vi "AttributeElementToString.vi"(8 "error in (no error)":errorcluster, 10 "attributeElement":T1, 11 "WriteAttribute in":refnum<class "XMLAttributeGenerator.lvclass">) -> (0 "error out":errorcluster, 2 "AttributeString":string, 3 "WriteAttribute out":refnum<class "XMLAttributeGenerator.lvclass">)   [LabVIEW 2016, in "XML.lvlib" / "XMLAttributeGenerator.lvclass"]
doc: "This method calls the format attribute method for a single attribute."
uses:
  <userlib>/Common/XML/XMLAttributeGenerator/XMLAttributeGenerator.lvclass
  <userlib>/Common/XML/Typedefs/AttributeElements.ctl
  <vilib>/dlg_ctls.llb/Space Constant.vi
  <userlib>/Common/XML/XML.lvlib
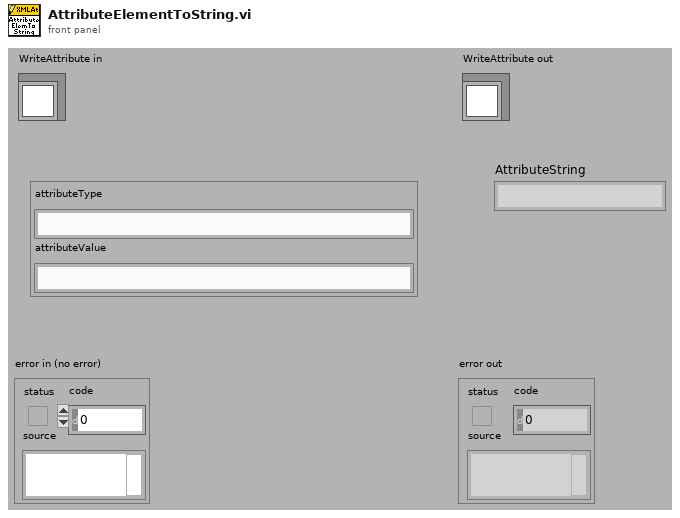
[diagram p1: front panel]
types:
  T1 = typedef "XML.lvlib/AttributeElements.ctl" = cluster{"attributeType":string, "attributeValue":string}
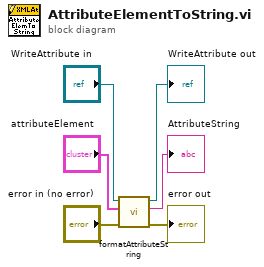
[diagram p0: block diagram]
diagram:
  n1 = call <userlib>:"formatAttributeString.vi"("error in (no error)"="error in (no error)", "attributeElement"="attributeElement", "WriteAttribute in"="WriteAttribute in") -> ("error out"=→"error out":errorcluster, "String"=→"AttributeString":string, "WriteAttribute out"=→"WriteAttribute out":refnum<class "XMLAttributeGenerator.lvclass">)  [unwired: 6 in]
